vi "ForkLiftDudeBro.vi"(11 "Buttons":T1) -> ()   [LabVIEW 2013]
uses:
  Utils/XBox Buttons.ctl
  Robot Global Data.vi
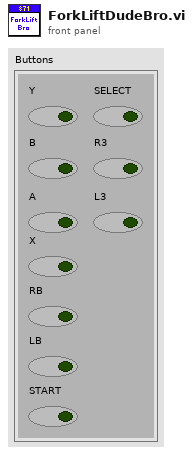
[diagram p1: front panel]
types:
  T1 = typedef "XBox Buttons.ctl" = cluster{"Y":bool, "B":bool, "A":bool, "X":bool, "RB":bool, "LB":bool, "START":bool, "SELECT":bool, "R3":bool, "L3":bool}
  T2 = typedef "WPI_MotorControlDeviceRef.ctl" = cluster{"DeviceStatus":errorcluster, "Type":enum16{"PWM", "CAN"}, "PWM":cluster{"Digital Module":T3, "PWM Channel":T4, "DeadBand":T5}, "CAN":cluster{"Device Number":u8, "Control Mode":T6, "Semaphore":T7, "Max Vout":dbl}, "Invert":bool, "TransformRef":T8, "InvTransformRef":T8}
  T3 = typedef "FPGA_TypedefDigitalModule.ctl" = enum16{"Digital Module 1", "Digital Module 2"}
  T4 = typedef "FPGA_DIOPWMChannel.ctl" = enum8{"PWM 1", "PWM 2", "PWM 3", "PWM 4", "PWM 5", "PWM 6", "PWM 7", "PWM 8", "PWM 9", "PWM 10", "Invalid"}
  T5 = typedef "WPI_PWMDeadband.ctl" = cluster{"Name":string, "maxPositivePwm":i32, "minPositivePwm":i32, "centerPwm":i32, "maxNegativePwm":i32, "minNegativePwm":i32, "angularRange":u16}
  T6 = typedef "WPI_CANJaguar_ControlMode.ctl" = enum8{"Percent VBus", "Current", "Speed", "Position", "Voltage"}
  T7 = typedef "Semaphore RefNum" = refnum<k1>
  T8 = typedef "WPI_PWMTransform_ConPane.ctl" = refnum<vi>
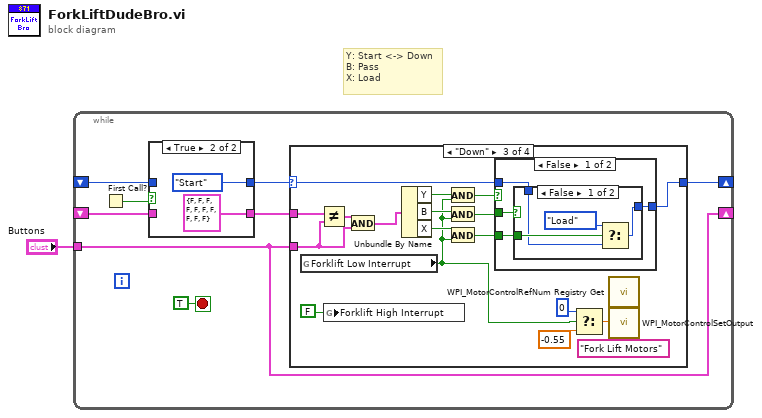
[diagram p0: block diagram]
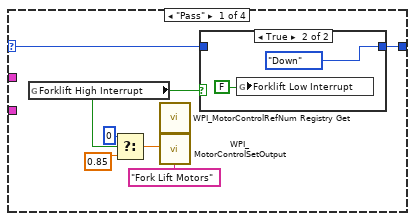
[diagram p3: hidden frame]
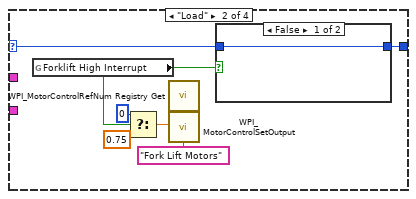
[diagram p5: hidden frame]
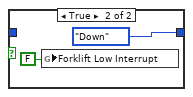
[diagram p6: hidden frame]
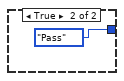
[diagram p7: hidden frame]
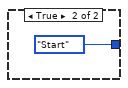
[diagram p8: hidden frame]
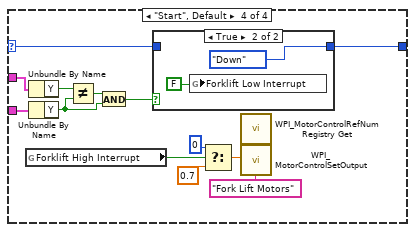
[diagram p9: hidden frame]
diagram:
  # "Y: Start <-> Down\nB: Pass\nX: Load"
  n1 = while {
    shift-right: [w6] -> _
    shift-left: _ -> [w7]
    tunnel: "Buttons" -> [w5]
    shift-right: [w5] -> _
    shift-left: _ -> [w3]
    stop <- TRUE stop-if-true
    n2 = First Call?() -> (First Call?: T/F=w8:bool)
    n3 = case shown="True" w8 {
      tunnel: [w11 enum16{"Pass", "Load", "Down", "Start"}."Start" ("Fork LIift Enum")] -> w9
      tunnel: w7 -> [w11 _]
      tunnel: [w10 T1 {"Y"=FALSE, "B"=FALSE, "A"=FALSE, "X"=FALSE, "RB"=FALSE, "LB"=FALSE, "START"=FALSE, "SELECT"=FALSE, "R3"=FALSE, "L3"=FALSE} ("Buttons")] -> w4
      tunnel: w3 -> [w10 _]
      frame False {
      }
      frame True {
      }
    }
    n4 = case shown="\"Down\"" w9 {
      selector: w9 -> [w22 w27 w55 w76]
      tunnel: [w21 w28 w56 w68] -> w6
      tunnel: w5 -> [_ _ w47 w82]
      tunnel: w4 -> [_ _ w57 w80]
      frame "Pass" {
        n5 = global read "Robot Global Data.vi" "Forklift High Interrupt"() -> (w14:bool)
        n6 = Select(t=0, s=w14, f=0.85) -> (s? t:f=w17:dbl)
        n7 = call <vilib>:"WPI_MotorControlRefNum Registry Get.vi"("refnum name"="Fork Lift Motors") -> ("error out"=w20:errorcluster, "MotorControlDevRef"=w19:T2)  [unwired: 9 in]
        n8 = call <vilib>:"WPI_MotorControlSetOutput.vi"("error in (no error)"=w20, "Output"=w17, "MotorControlDevRef"=w19) -> ()  [unwired: 6 in, 3 out]
        n9 = case shown="True" w14 {
          tunnel: w22 -> [w23 _]
          tunnel: [w23 enum16{"Pass", "Load", "Down", "Start"}."Down" ("Fork LIift Enum")] -> w21
          frame False {
          }
          frame True {
            n10 = global write "Robot Global Data.vi" "Forklift Low Interrupt"(FALSE) -> ()
          }
        }
      }
      frame "Load" {
        n11 = global read "Robot Global Data.vi" "Forklift High Interrupt"() -> (w26:bool)
        n12 = Select(t=0, s=w26, f=0.75) -> (s? t:f=w32:dbl)
        n13 = call <vilib>:"WPI_MotorControlRefNum Registry Get.vi"("refnum name"="Fork Lift Motors") -> ("error out"=w29:errorcluster, "MotorControlDevRef"=w30:T2)  [unwired: 9 in]
        n14 = call <vilib>:"WPI_MotorControlSetOutput.vi"("error in (no error)"=w29, "Output"=w32, "MotorControlDevRef"=w30) -> ()  [unwired: 6 in, 3 out]
        n15 = case shown="False" w26 {
          tunnel: [w35 enum16{"Pass", "Load", "Down", "Start"}."Down" ("Fork LIift Enum")] -> w28
          tunnel: w27 -> [w35 _]
          frame False {
          }
          frame True {
            n16 = global write "Robot Global Data.vi" "Forklift Low Interrupt"(FALSE) -> ()
          }
        }
      }
      frame "Down" {
        n17 = global read "Robot Global Data.vi" "Forklift Low Interrupt"() -> (w38:bool)
        n18 = Not Equal?(x=w57, y=w47) -> (x != y?=w48:T1)
        n19 = global write "Robot Global Data.vi" "Forklift High Interrupt"(FALSE) -> ()
        n20 = And(x=w48, y=w47) -> (x .and. y?=w40:T1)
        n21 = Unbundle By Name(w40) -> ("Y"=w45:bool, "B"=w44:bool, "X"=w42:bool)
        n22 = And(x=w45, y=w38) -> (x .and. y?=w46:bool)
        n23 = And(x=w44, y=w38) -> (x .and. y?=w43:bool)
        n24 = And(x=w42, y=w38) -> (x .and. y?=w41:bool)
        n25 = case shown="False" w46 {
          tunnel: [w60 enum16{"Pass", "Load", "Down", "Start"}."Start" ("Fork LIift Enum")] -> w56
          tunnel: w43 -> [w61 _]
          tunnel: w55 -> [w59 _]
          tunnel: w41 -> [w58 _]
          frame False {
            n26 = case shown="False" w61 {
              tunnel: [w62 enum16{"Pass", "Load", "Down", "Start"}."Pass" ("Fork LIift Enum")] -> w60
              tunnel: w59 -> [w64 _]
              tunnel: w58 -> [w65 _]
              frame False {
                n27 = Select(t=enum16{"Pass", "Load", "Down", "Start"}."Load" ("Fork LIift Enum"), s=w65, f=w64) -> (s? t:f=w62:enum16{"Pass", "Load", "Down", "Start"})
              }
              frame True {
              }
            }
          }
          frame True {
          }
        }
        n28 = Select(t=0, s=w38, f=-0.55) -> (s? t:f=w53:dbl)
        n29 = call <vilib>:"WPI_MotorControlRefNum Registry Get.vi"("refnum name"="Fork Lift Motors") -> ("error out"=w54:errorcluster, "MotorControlDevRef"=w49:T2)  [unwired: 9 in]
        n30 = call <vilib>:"WPI_MotorControlSetOutput.vi"("error in (no error)"=w54, "Output"=w53, "MotorControlDevRef"=w49) -> ()  [unwired: 6 in, 3 out]
      }
      frame "Start", Default {
        n31 = global read "Robot Global Data.vi" "Forklift High Interrupt"() -> (w69:bool)
        n32 = Unbundle By Name(w80) -> ("Y"=w79:bool)
        n33 = Unbundle By Name(w82) -> ("Y"=w78:bool)
        n34 = Not Equal?(x=w79, y=w78) -> (x != y?=w81:bool)
        n35 = And(x=w81, y=w78) -> (x .and. y?=w77:bool)
        n36 = case shown="True" w77 {
          tunnel: [w83 enum16{"Pass", "Load", "Down", "Start"}."Down" ("Fork LIift Enum")] -> w68
          tunnel: w76 -> [w83 _]
          frame False {
          }
          frame True {
            n37 = global write "Robot Global Data.vi" "Forklift Low Interrupt"(FALSE) -> ()
          }
        }
        n38 = Select(t=0, s=w69, f=0.7) -> (s? t:f=w72:dbl)
        n39 = call <vilib>:"WPI_MotorControlRefNum Registry Get.vi"("refnum name"="Fork Lift Motors") -> ("error out"=w75:errorcluster, "MotorControlDevRef"=w74:T2)  [unwired: 9 in]
        n40 = call <vilib>:"WPI_MotorControlSetOutput.vi"("error in (no error)"=w75, "Output"=w72, "MotorControlDevRef"=w74) -> ()  [unwired: 6 in, 3 out]
      }
    }
  }
